vi "Set-image-type-menu.vi"(7 "Menu ref.":refnum<k9>, 8 "error in (no error)":errorcluster, 10 "Image type":T1, 11 "UI ref. in":refnum<data-value>) -> (0 "error out":errorcluster, 3 "UI ref.":refnum<data-value>)   [LabVIEW 2013, in "CameraVision.lvlib" / "CV-UI.lvclass"]
uses:
  CV-UI.lvclass
  Image-selector.ctl
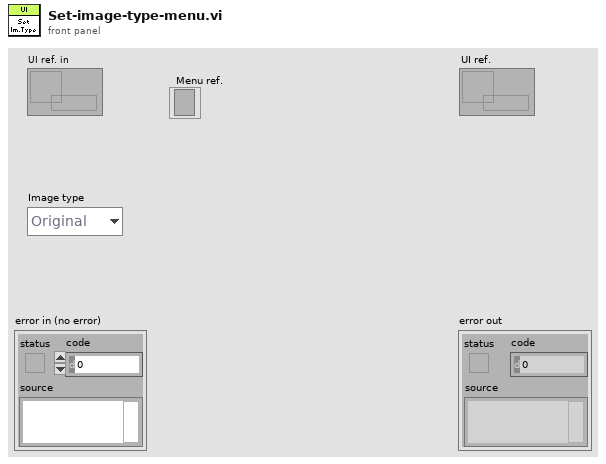
[diagram p1: front panel]
types:
  T1 = typedef "CameraVision.lvlib/CV-UI.lvclass/Image-selector.ctl" = enum16{"Original", "Corrected", "Binary"}
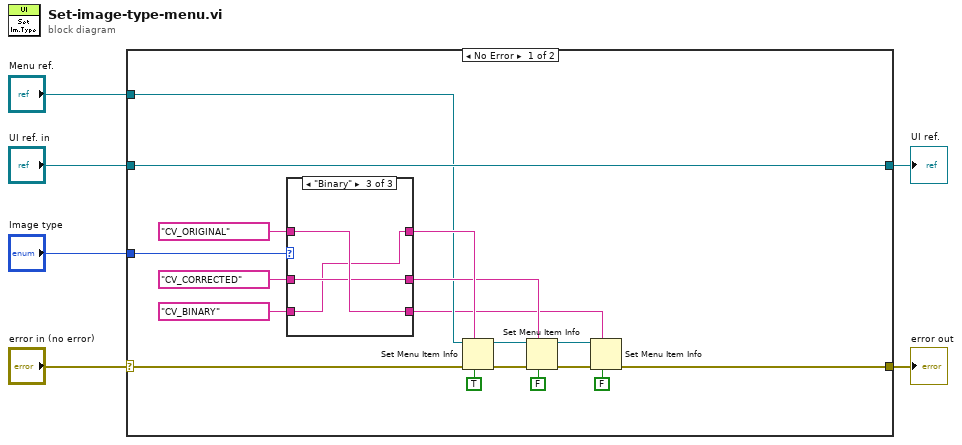
[diagram p0: block diagram]
diagram:
  n1 = case shown="No Error" "error in (no error)" {
    selector: "error in (no error)" -> [w17 w35]
    tunnel: [w9 w35] -> w5
    tunnel: "UI ref. in" -> [w14 w34]
    tunnel: [w14 w34] -> w3
    tunnel: "Image type" -> [w20 _]
    tunnel: "Menu ref." -> [w13 _]
    frame No Error {
      n2 = case shown="\"Binary\"" w20 {
        tunnel: "CV_ORIGINAL" ("item tag") -> [w26 w30 w33]
        tunnel: "CV_CORRECTED" ("item tag") -> [w27 w29 w32]
        tunnel: [w27 w30 w32] -> w15
        tunnel: [w26 w29 w31] -> w16
        tunnel: "CV_BINARY" ("item tag") -> [w25 w28 w31]
        tunnel: [w25 w28 w33] -> w8
        frame "Original", Default {
        }
        frame "Corrected" {
        }
        frame "Binary" {
        }
      }
      n3 = Set Menu Item Info(6:TRUE ("checked"), 7:w16, 8:w17, 11:w13) -> (0:w21:errorcluster, 3:w24:refnum<k9>)  [unwired: 3 in]
      n4 = Set Menu Item Info(6:FALSE ("checked"), 7:w15, 8:w21, 11:w24) -> (0:w10:errorcluster, 3:w7:refnum<k9>)  [unwired: 3 in]
      n5 = Set Menu Item Info(6:FALSE ("checked"), 7:w8, 8:w10, 11:w7) -> (0:w9:errorcluster)  [unwired: 3 in, 1 out]
    }
    frame Error {
    }
  }
  "error out" <- w5
  "UI ref." <- w3
